vi "DMK Dev tool.vi"() -> ()   [LabVIEW 2018]
uses:
  builds/Camera.lvlibp/Camera.lvclass
panel:
  in  "Sharpness":dbl
  in  "Gamma":dbl
  in  "Gain":dbl
  in  "Exposure":dbl
  out "error out":errorcluster
  in  "Brightness":dbl
  in  "stop":bool
  out "Image":T1(plugin-control)
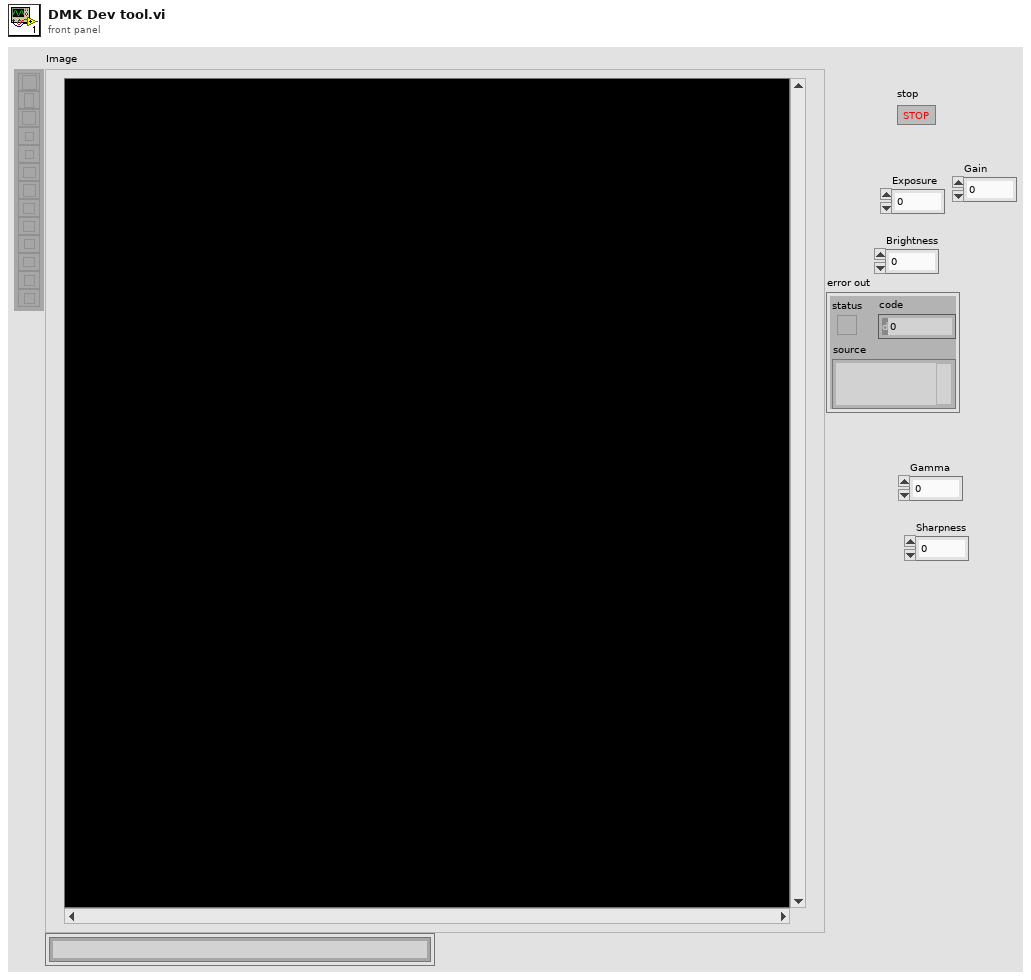
[diagram p1: front panel]
types:
  T1 = typedef "IMAQ Image.ctl" = refnum<image>
  T2 = typedef "Camera.lvlibp/IMAQ Image.ctl" = refnum<image>
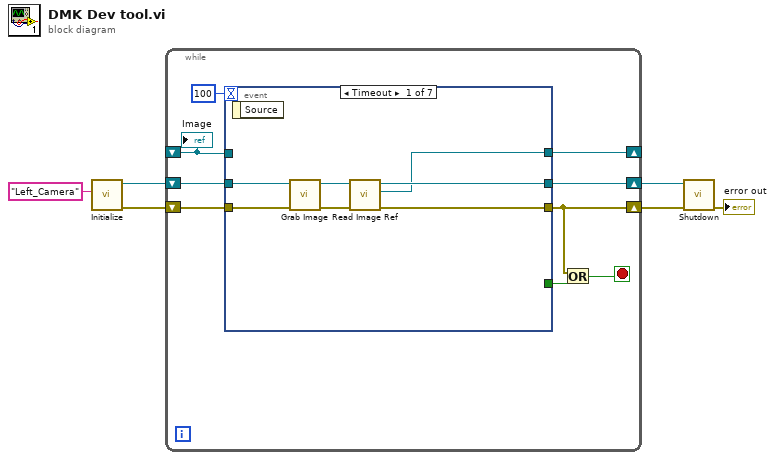
[diagram p0: block diagram]
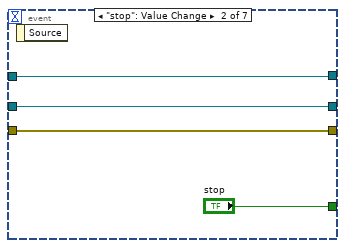
[diagram p2: hidden frame]
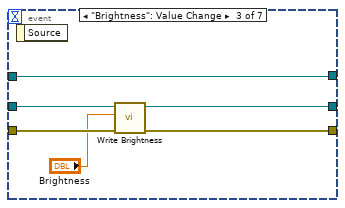
[diagram p3: hidden frame]
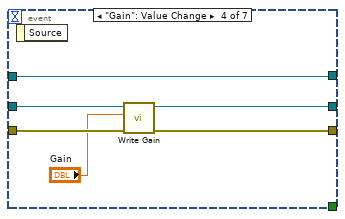
[diagram p4: hidden frame]
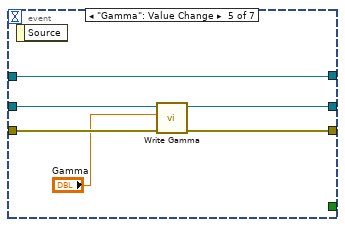
[diagram p5: hidden frame]
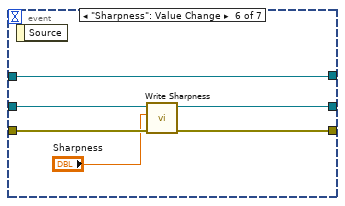
[diagram p6: hidden frame]
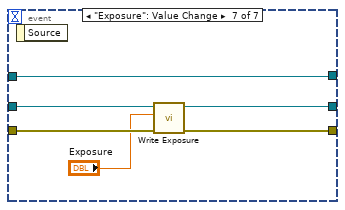
[diagram p7: hidden frame]
diagram:
  n1 = call "Initialize.vi"("Device"="Left_Camera") -> ("error out"=w4:errorcluster, "Camera out"=w6:refnum<class "Camera.lvclass">)  [unwired: 9 in]
  n2 = while {
    shift-right: [w13] -> w2
    shift-left: w6 -> [w15]
    shift-right: [w9] -> w3
    shift-left: w4 -> [w14]
    shift-right: [w12] -> _
    shift-left: _ -> [w11]
    stop <- w8 stop-if-true
    n3 = event shown="[0] Timeout" {
      selector: _ -> [_ _ _ _ _ _ _]
      dyn-events: _ -> [_ _ _ _ _ _ _]
      timeout: 100 -> [_ _ _ _ _ _ _]
      tunnel: w15 -> [w22 w26 w30 w37 w43 w49 w55]
      tunnel: w14 -> [w21 w25 w31 w36 w42 w48 w52]
      tunnel: [w18 w26 w29 w35 w41 w46 w54] -> w13
      tunnel: [w17 w25 w28 w34 w40 w47 w53] -> w9
      tunnel: [w16 w24 w32 w38 w44 w50 w56] -> w12
      tunnel: w11 -> [_ w24 w32 w38 w44 w50 w56]
      tunnel: [_ "stop" _ _ _ _ _] -> w10
      event Timeout {
        n4 = event-data() -> ()  [unwired: 1 in, 1 out]
        n5 = call-dynamic "Grab Image.vi"("error in (no error)"=w21, "Camera in"=w22) -> ("error out"=w20:errorcluster, "Camera out"=w19:refnum<class "Camera.lvclass">)  [unwired: 8 in]
        n6 = call "Read Image Ref.vi"("error in (no error)"=w20, "Camera in"=w19) -> ("error out"=w17:errorcluster, "Image"=w16:T2, "Camera out"=w18:refnum<class "Camera.lvclass">)  [unwired: 7 in]
      }
      event "stop": Value Change {
        n7 = event-data() -> ()  [unwired: 1 in, 1 out]
      }
      event "Brightness": Value Change {
        n8 = event-data() -> ()  [unwired: 1 in, 1 out]
        n9 = call "Write Brightness.vi"("error in"=w31, "Brightness"="Brightness", "Camera in"=w30) -> ("error out"=w28:errorcluster, "Camera out"=w29:refnum<class "Camera.lvclass">)  [unwired: 7 in]
      }
      event "Gain": Value Change {
        n10 = event-data() -> ()  [unwired: 1 in, 1 out]
        n11 = call "Write Gain.vi"("error in (no error)"=w36, "Gain"="Gain", "Camera in"=w37) -> ("error out"=w34:errorcluster, "Camera out"=w35:refnum<class "Camera.lvclass">)  [unwired: 7 in]
      }
      event "Gamma": Value Change {
        n12 = event-data() -> ()  [unwired: 1 in, 1 out]
        n13 = call "Write Gamma.vi"("error in (no error)"=w42, "Gamma"="Gamma", "Camera in"=w43) -> ("error out"=w40:errorcluster, "Camera out"=w41:refnum<class "Camera.lvclass">)  [unwired: 7 in]
      }
      event "Sharpness": Value Change {
        n14 = event-data() -> ()  [unwired: 1 in, 1 out]
        n15 = call "Write Sharpness.vi"("error in"=w48, "Sharpness"="Sharpness", "Camera in"=w49) -> ("error out"=w47:errorcluster, "Camera out"=w46:refnum<class "Camera.lvclass">)  [unwired: 7 in]
      }
      event "Exposure": Value Change {
        n16 = event-data() -> ()  [unwired: 1 in, 1 out]
        n17 = call "Write Exposure.vi"("error in (no error)"=w52, "Exposure"="Exposure", "Camera in"=w55) -> ("error out"=w53:errorcluster, "Camera out"=w54:refnum<class "Camera.lvclass">)  [unwired: 7 in]
      }
    }
    n18 = Or(x=w9, y=w10) -> (x .or. y?=w8:bool)
    "Image" <- w11
  }
  n19 = call "Shutdown.vi"("error in"=w3, "Camera in"=w2) -> ("error out"=→"error out":errorcluster)  [unwired: 8 in, 1 out]
